vi "Best fit circle.vi"(0 "x array":dbl[](array[numeric]), 1 "y array":dbl[](array[numeric])) -> (2 "x centre":dbl, 3 "y centre":dbl, 4 "radius":dbl)   [LabVIEW 2014]
doc: "Finds the best fit circle using a least squares method. Input arrays (corresponding values of x and y) must have a minimum of 3 values each"
uses:
  <vilib>/Analysis/baseanly.llb/Real A x B.vi
  <vilib>/Analysis/baseanly.llb/A x Vector.vi
  <vilib>/Analysis/baseanly.llb/Real Inverse Matrix.vi
  <vilib>/Analysis/Matrix/Numeric/Conversions/Array To Matrix - RA2.vi
  <vilib>/Analysis/Matrix/NI_Matrix.lvlib
  <vilib>/Analysis/NI_AALBase.lvlib
panel:
  # "Paul Nathan 23/06/2015"
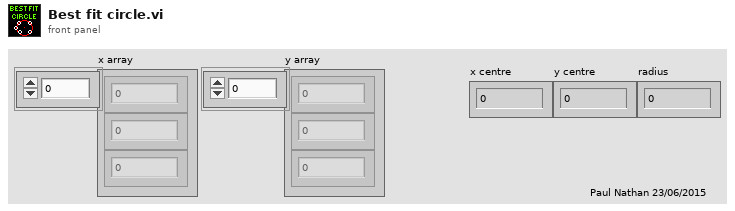
[diagram p1: front panel]
types:
  T1 = typedef "NI_Matrix.lvlib/RealMatrix.ctl" = dbl[][]
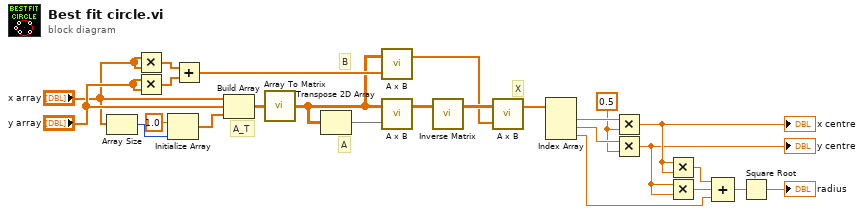
[diagram p0: block diagram]
diagram:
  w10 = 0.5 ("y")
  # "A_T"
  # "X"
  # "A"
  # "B"
  n1 = Array Size(array="x array") -> (size(s)=w25:i32)
  n2 = Multiply(x="x array", y="x array") -> (x*y=w21:dbl[])
  n3 = Multiply(x="y array", y="y array") -> (x*y=w22:dbl[])
  n4 = Initialize Array(1.0 ("element"), w25) -> (w23:dbl[])
  n5 = Add(x=w21, y=w22) -> (x+y=w14:dbl[])
  n6 = Build Array("x array", "y array", w23) -> (w18:dbl[][])
  n7 = call-poly <vilib>:"Array To Matrix.vi"("Real 2D Array"=w18) -> ("Real Matrix"=w1:T1)
  n8 = Transpose 2D Array(2D array=w1) -> (transposed array=w2:T1)
  n9 = call-poly <vilib>:"A x B.vi"("Vector"=w14, "A"=w1) -> ("A x Vector"=w15:dbl[])  [unwired: 1 out]
  n10 = call-poly <vilib>:"A x B.vi"("B"=w2, "A"=w1) -> ("A x B"=w17:T1)  [unwired: 1 out]
  n11 = call-poly <vilib>:"Inverse Matrix.vi"("Input Matrix"=w17) -> ("Inverse Matrix"=w16:T1)  [unwired: 1 in, 1 out]
  n12 = call-poly <vilib>:"A x B.vi"("Vector"=w15, "A"=w16) -> ("A x Vector"=w13:dbl[])  [unwired: 1 out]
  n13 = Index Array(array=w13) -> (element #1=w12:dbl, element #2=w11:dbl, element #3=w5:dbl)  [unwired: 3 in]
  n14 = Multiply(x=w12, y=w10) -> (x*y=w9:dbl)
  "x centre" <- w9
  n15 = Multiply(x=w11, y=w10) -> (x*y=w8:dbl)
  "y centre" <- w8
  n16 = Multiply(x=w9, y=w9) -> (x*y=w7:dbl)
  n17 = Multiply(x=w8, y=w8) -> (x*y=w6:dbl)
  n18 = Compound Arithmetic op=ADD(w7, w6, w5) -> (w4:dbl)
  n19 = Square Root(x=w4) -> (sqrt(x)=→"radius":dbl)
